vi "Experiment01.vi"() -> ()   [LabVIEW 2009]
uses:
  <vilib>/imath/engines/lvmath2/RunTimeEngine/ErrorHandling/NIMS_Finalize Error.vi
  <vilib>/imath/engines/lvmath2/RunTimeEngine/Parser/MC_Version.vi
  <vilib>/imath/engines/lvmath2/RunTimeEngine/NodeEndStatement/NIMS_NodeEndStatement_Output.vi
  <instcachedir>/0/NIMS_NodeEndStatement_Output_B70DDD75627E4997AAE11E9955EDAA25.lvgen/NIMS_NodeEndStatement_Output_B70DDD75627E4997AAE11E9955EDAA25_002.vi
  <instcachedir>/0/NIMS_NodeEndStatement_Output_B70DDD75627E4997AAE11E9955EDAA25.lvgen/NIMS_NodeEndStatement_Output_B70DDD75627E4997AAE11E9955EDAA25_003.vi
  <vilib>/imath/engines/lvmath/Functions/Error Handling/MergeErrorsWrapper.vi
  <instcachedir>/0/NIMS_NodeEndStatement_Output_B70DDD75627E4997AAE11E9955EDAA25.lvgen/NIMS_NodeEndStatement_Output_B70DDD75627E4997AAE11E9955EDAA25_001.vi
  <vilib>/imath/engines/lvmath2/RunTimeEngine/Managers/WorkSpace/UID Generator.vi
  <vilib>/imath/engines/lvmath/Functions/Error Handling/error.ctl
  <instcachedir>/0/NIMS_NodeEndStatement_Output_B70DDD75627E4997AAE11E9955EDAA25.lvgen/NIMS_NodeEndStatement_Output_B70DDD75627E4997AAE11E9955EDAA25_000.vi
  <vilib>/imath/engines/lvmath2/RunTimeEngine/Managers/SymbolTable/Clear UID.vi
  <vilib>/imath/engines/lvmath2/RunTimeEngine/VariableToken/NIMS_VariableToken_CondDefined.vi
  <instcachedir>/0/NIMS_VariableToken_CondDefined_5641E79000FB4D628475532441475385.lvgen/NIMS_VariableToken_CondDefined_5641E79000FB4D628475532441475385_001.vi
  <vilib>/imath/engines/lvmath/Functions/Error Handling/MC_Mask_Errors.vi
  <vilib>/imath/engines/lvmath2/RunTimeEngine/BuiltInFunctions/rem/NIMS_rem_no checks.vi
  <instcachedir>/0/NIMS_rem_no checks_4CC9B305AB7E42EF90AFC4973FB32F8D.lvgen/NIMS_rem_no checks_4CC9B305AB7E42EF90AFC4973FB32F8D_000.vi
  <vilib>/imath/engines/lvmath2/RunTimeEngine/BuiltInFunctions/uint32/NIMS_uint32(real).vi
  <instcachedir>/0/NIMS_uint32(real)_FDC83D68D45943DDB8F3F934FF8A712F.lvgen/NIMS_uint32(real)_FDC83D68D45943DDB8F3F934FF8A712F_000.vi
  <vilib>/imath/engines/lvmath2/RunTimeEngine/BuiltInFunctions/double/NIMS_double.vi
  <instcachedir>/0/NIMS_double_2CE444F3CE4146B199A482FE12545E45.lvgen/NIMS_double_2CE444F3CE4146B199A482FE12545E45_000.vi
  <vilib>/imath/engines/lvmath2/RunTimeEngine/RangeToken/NIMS_Range.vi
  <instcachedir>/0/NIMS_Range_6D647EC16A744C98B5DE1D649A2D648D.lvgen/NIMS_Range_6D647EC16A744C98B5DE1D649A2D648D_001.vi
  <vilib>/imath/engines/lvmath2/RunTimeEngine/BuiltInFunctions/length/NIMS_length(GV).vi
  <instcachedir>/0/NIMS_length(GV)_7D6E94E728E145E68721C53861296D96.lvgen/NIMS_length(GV)_7D6E94E728E145E68721C53861296D96_000.vi
  <instcachedir>/0/NIMS_Range_6D647EC16A744C98B5DE1D649A2D648D.lvgen/NIMS_Range_6D647EC16A744C98B5DE1D649A2D648D_000.vi
  <vilib>/imathl/engines/lvmath/Functions/Error Handling/Create Error.vi
  <vilib>/imath/engines/lvmath2/RunTimeEngine/ReplaceToken/NIMS_Replace - V(S)=S.vi
  <instcachedir>/0/NIMS_Replace - V(S)=S_670A9E0533664C1D848C8E58B3321B6A.lvgen/NIMS_Replace - V(S)=S_670A9E0533664C1D848C8E58B3321B6A_002.vi
  <vilib>/imath/engines/lvmath2/RunTimeEngine/ReplaceToken/NIMS_Replace - Size Check _(_)=S.vi
  <instcachedir>/0/NIMS_Replace - Size Check _(_)=S_8596181D73404097BAB9CBB006194BB0.lvgen/NIMS_Replace - Size Check _(_)=S_8596181D73404097BAB9CBB006194BB0_002.vi
  <vilib>/imath/engines/lvmath2/RunTimeEngine/ReplaceToken/NIMS_Replace - Check Linear.vi
  <instcachedir>/0/NIMS_Replace - Check Linear_9243CBB174894FF6977027453DA6955E.lvgen/NIMS_Replace - Check Linear_9243CBB174894FF6977027453DA6955E_002.vi
  <vilib>/imath/engines/lvmath2/RunTimeEngine/VariableToken/NIMS_VariableToken_CondDefinedDefinedByReplace.vi
  <instcachedir>/0/NIMS_VariableToken_CondDefinedDefinedByReplace_D162CFFC24174562A9FEA619A91E1A56.lvgen/NIMS_VariableToken_CondDefinedDefinedByReplace_D162CFFC24174562A9FEA619A91E1A56_002.vi
  <vilib>/imath/engines/lvmath2/RunTimeEngine/CommandStatement/MC_CommandStatement_break.vi
  <vilib>/imath/engines/lvmath2/RunTimeEngine/LocalVariableDefStatement/MC_LocalVariableDefStatement_Display.vi
  <vilib>/imath/engines/lvmath2/RunTimeEngine/RunTimeType/NIMS_RunTimeType_From StrictType (excl LVString).vi
  <vilib>/imath/engines/lvmath2/RunTimeEngine/ArithmeticOperatorToken/NIMS_ArithmeticOperator_times.vi
  <instcachedir>/0/NIMS_ArithmeticOperator_times_3987BC660D7947CD8628C10658A43225.lvgen/NIMS_ArithmeticOperator_times_3987BC660D7947CD8628C10658A43225_001.vi
  <instcachedir>/0/NIMS_ArithmeticOperator_times_3987BC660D7947CD8628C10658A43225.lvgen/NIMS_ArithmeticOperator_times_3987BC660D7947CD8628C10658A43225_000.vi
  <vilib>/imath/engines/lvmath2/RunTimeEngine/VariableToken/Read/NIMS_Get Elements - RV(_) - Check.vi
  <instcachedir>/0/NIMS_Get Elements - RV(_) - Check_60F12861D0564803969A5D0D0D1716CD.lvgen/NIMS_Get Elements - RV(_) - Check_60F12861D0564803969A5D0D0D1716CD_000.vi
  <instcachedir>/0/NIMS_VariableToken_CondDefined_5641E79000FB4D628475532441475385.lvgen/NIMS_VariableToken_CondDefined_5641E79000FB4D628475532441475385_000.vi
  <instcachedir>/0/NIMS_VariableToken_CondDefined_5641E79000FB4D628475532441475385.lvgen/NIMS_VariableToken_CondDefined_5641E79000FB4D628475532441475385_003.vi
  <vilib>/imath/engines/lvmath2/RunTimeEngine/BuiltInFunctions/abs/NIMS_abs(signed).vi
  <instcachedir>/0/NIMS_abs(signed)_C4FCB8E6058B49B797C7C8D53CA5F6EC.lvgen/NIMS_abs(signed)_C4FCB8E6058B49B797C7C8D53CA5F6EC_000.vi
  <instcachedir>/0/NIMS_Replace - V(S)=S_670A9E0533664C1D848C8E58B3321B6A.lvgen/NIMS_Replace - V(S)=S_670A9E0533664C1D848C8E58B3321B6A_001.vi
  <instcachedir>/0/NIMS_Replace - Size Check _(_)=S_8596181D73404097BAB9CBB006194BB0.lvgen/NIMS_Replace - Size Check _(_)=S_8596181D73404097BAB9CBB006194BB0_001.vi
  <instcachedir>/0/NIMS_Replace - Check Linear_9243CBB174894FF6977027453DA6955E.lvgen/NIMS_Replace - Check Linear_9243CBB174894FF6977027453DA6955E_001.vi
  <instcachedir>/0/NIMS_VariableToken_CondDefinedDefinedByReplace_D162CFFC24174562A9FEA619A91E1A56.lvgen/NIMS_VariableToken_CondDefinedDefinedByReplace_D162CFFC24174562A9FEA619A91E1A56_001.vi
  <instcachedir>/0/NIMS_Replace - V(S)=S_670A9E0533664C1D848C8E58B3321B6A.lvgen/NIMS_Replace - V(S)=S_670A9E0533664C1D848C8E58B3321B6A_000.vi
  <instcachedir>/0/NIMS_Replace - Size Check _(_)=S_8596181D73404097BAB9CBB006194BB0.lvgen/NIMS_Replace - Size Check _(_)=S_8596181D73404097BAB9CBB006194BB0_000.vi
  <instcachedir>/0/NIMS_Replace - Check Linear_9243CBB174894FF6977027453DA6955E.lvgen/NIMS_Replace - Check Linear_9243CBB174894FF6977027453DA6955E_000.vi
  <instcachedir>/0/NIMS_VariableToken_CondDefinedDefinedByReplace_D162CFFC24174562A9FEA619A91E1A56.lvgen/NIMS_VariableToken_CondDefinedDefinedByReplace_D162CFFC24174562A9FEA619A91E1A56_000.vi
  <vilib>/imath/engines/lvmath2/RunTimeEngine/Managers/SymbolTable/NIMS_WorkSpace.lvlib
panel:
  out "Current VI path 11":string
  out "New Path for Picture 11":string
  out "Part Stripped 11":string
  out "Stripped Path 11":string
  out "Current VI path 10":string
  out "New Path for Picture 10":string
  out "Part Stripped 10":string
  out "Stripped Path 10":string
  out "Current VI path 9":string
  out "New Path for Picture 9":string
  out "Part Stripped 9":string
  out "Stripped Path 9":string
  out "Current VI path 8":string
  out "New Path for Picture 8":string
  out "Part Stripped 8":string
  out "Stripped Path 8":string
  out "Current VI path 7":string
  out "New Path for Picture 7":string
  out "Part Stripped 7":string
  out "Stripped Path 7":string
  out "Current VI path 6":string
  out "New Path for Picture 6":string
  out "Part Stripped 6":string
  out "Stripped Path 6":string
  out "Current VI path 5":string
  out "New Path for Picture 5":string
  out "Part Stripped 5":string
  out "Stripped Path 5":string
  out "Current VI path 4":string
  out "New Path for Picture 4":string
  out "Part Stripped 4":string
  out "Stripped Path 4":string
  out "Current VI path 3":string
  out "New Path for Picture 3":string
  out "Part Stripped 3":string
  out "Stripped Path 3":string
  out "Current VI path 2":string
  out "New Path for Picture 2":string
  out "Part Stripped 2":string
  out "Stripped Path 2":string
  out "Current VI path":string
  out "New Path for Picture":string
  out "Part Stripped":string
  out "Stripped Path":string
  out "error out":errorcluster
  in  "2.TECNIQUE USED TO CALCULATE VSWR":bool
  out "error out":errorcluster
  in  "1.TECNIQUE USED TO CALCULATE VSWR":bool
  out "?":errorcluster
  out "?":errorcluster
  in  "?":T1(tab)
  out "?":dbl[](graph)
  out "Characteristic Impedance":dbl
  out "Voltage 2":dbl
  out "Distance(Meter)":dbl
  in  "Slide":dbl(slide) scale=0.0..0.3
  out "?":errorcluster
  in  "HELP FOR SLOTTED LINE":bool
  out "error out":errorcluster
  out "?":dbl[](graph)
  out "VSWR Meter":dbl(knob) caption="Meter" scale=500.0..1.0 scale format="%#_10g"
  out "Ideal VSWR":dbl
  in  "?":enum32{"LOADS"}(tab)
  in  "Type of Loads":T2(radio)
  out "Resistance":dbl
  out "Reactance":dbl
  in  "Resistance":dbl(slide) scale=0.0..1000.0
  in  "Reactance":dbl(slide) scale=0.0..1000.0
  out "?":errorcluster
  in  "HELP FOR LOADS":bool
  out "error out":errorcluster
  in  "?":enum32{"ATTENUATOR"}(tab)
  out "?":dbl[](graph)
  in  "Set the value of attenuation in dB":dbl(slide) scale=0.0..100.0
  out "?":errorcluster
  in  "HELP FOR ATTENUATOR":bool
  out "error out":errorcluster
  in  "?":enum32{"ISOLATOR"}(tab)
  out "?":dbl[](graph)
  in  "?":bool
  out "?":errorcluster
  in  "HELP FOR ISOLATOR":bool
  out "error out":errorcluster
  in  "?":enum32{"MODULATOR"}(tab)
  in  "Modulating Frequency(KHz)":dbl(slide) scale=0.5..1.5
  out "?":errorcluster
  out "?":dbl[](graph)
  in  "HELP FOR MODULATOR":bool
  out "error out":errorcluster
  in  "?":enum32{"SOURCE"}(tab)
  out "?":dbl[](graph)
  in  "Frequency of carrier wave(GHz)":dbl(slide) scale=8.0..15.0
  in  "Voltage":dbl(knob) scale=0.0..20.0 scale format="%#_10g"
  out "?":errorcluster
  in  "HELP FOR SOURCE":bool
  out "error out":errorcluster
  # "Backward Direction"
  # "Forward direction"
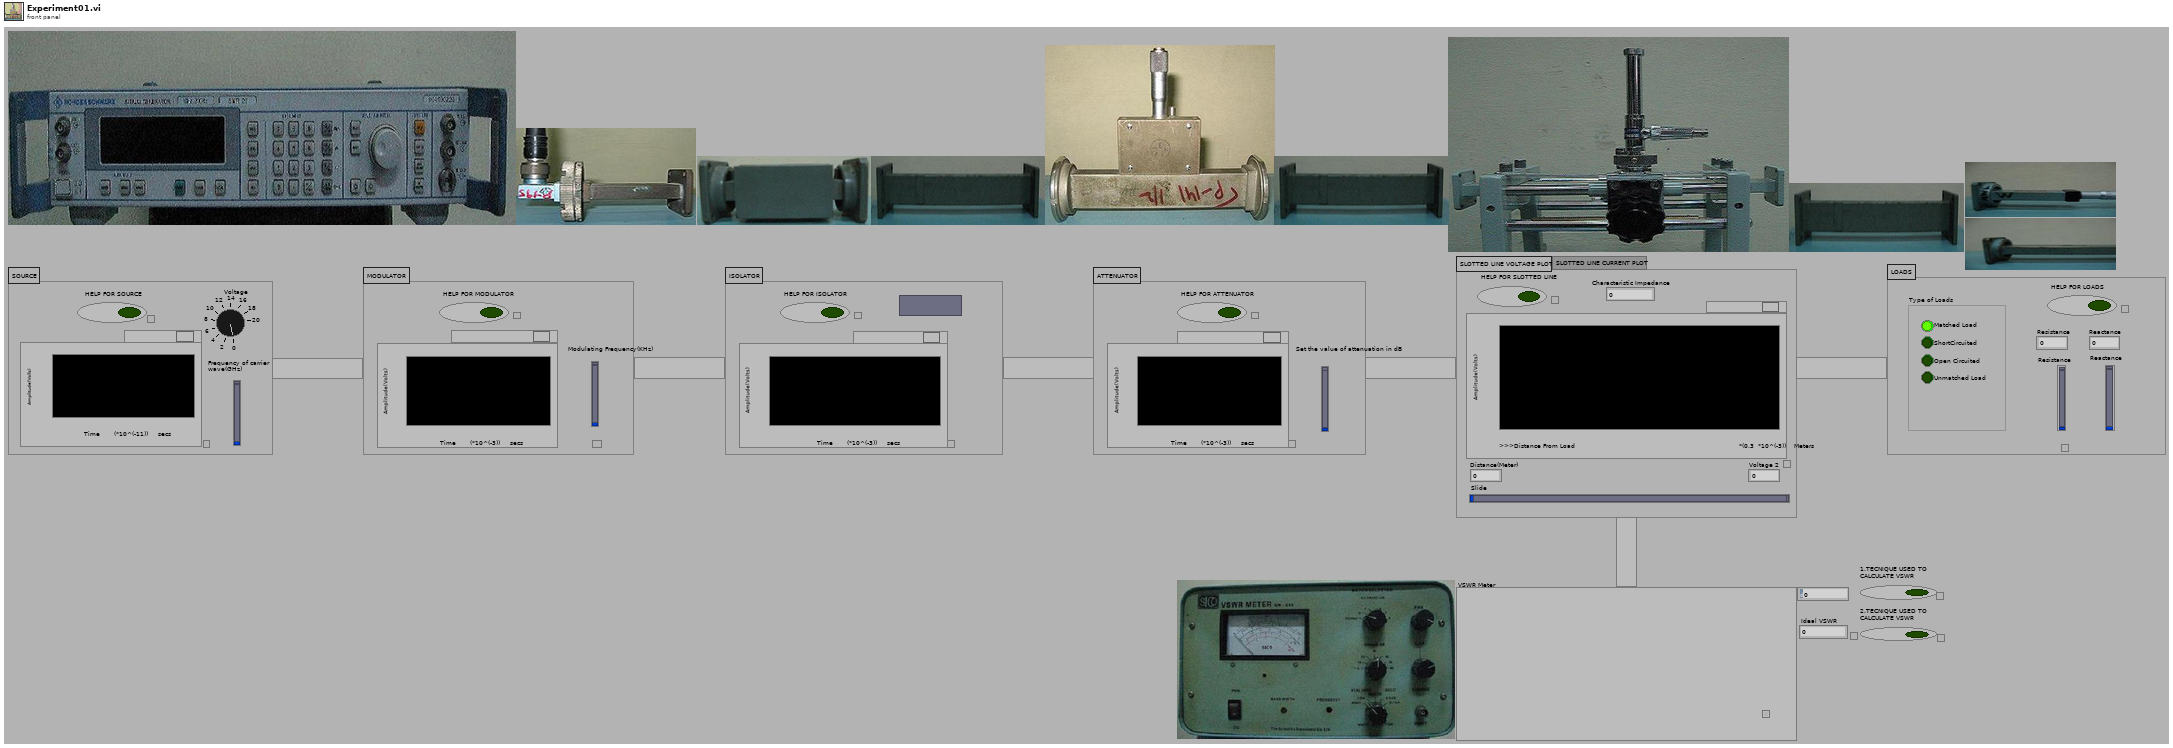
[diagram p1: front panel]
types:
  T1 = enum32{"SLOTTED LINE VOLTAGE PLOT", "SLOTTED LINE CURRENT PLOT"}
  T2 = enum32{"Matched Load", "ShortCircuited", "Open Circuited", "Unmatched Load"}
  T3 = typedef "imagedata.ctl" = cluster{"image type":i32, "image depth":i32, "image":u8[], "mask":u8[], "colors":u32[], "Rectangle":cluster{"left":i16, "top":i16, "right":i16, "bottom":i16}}
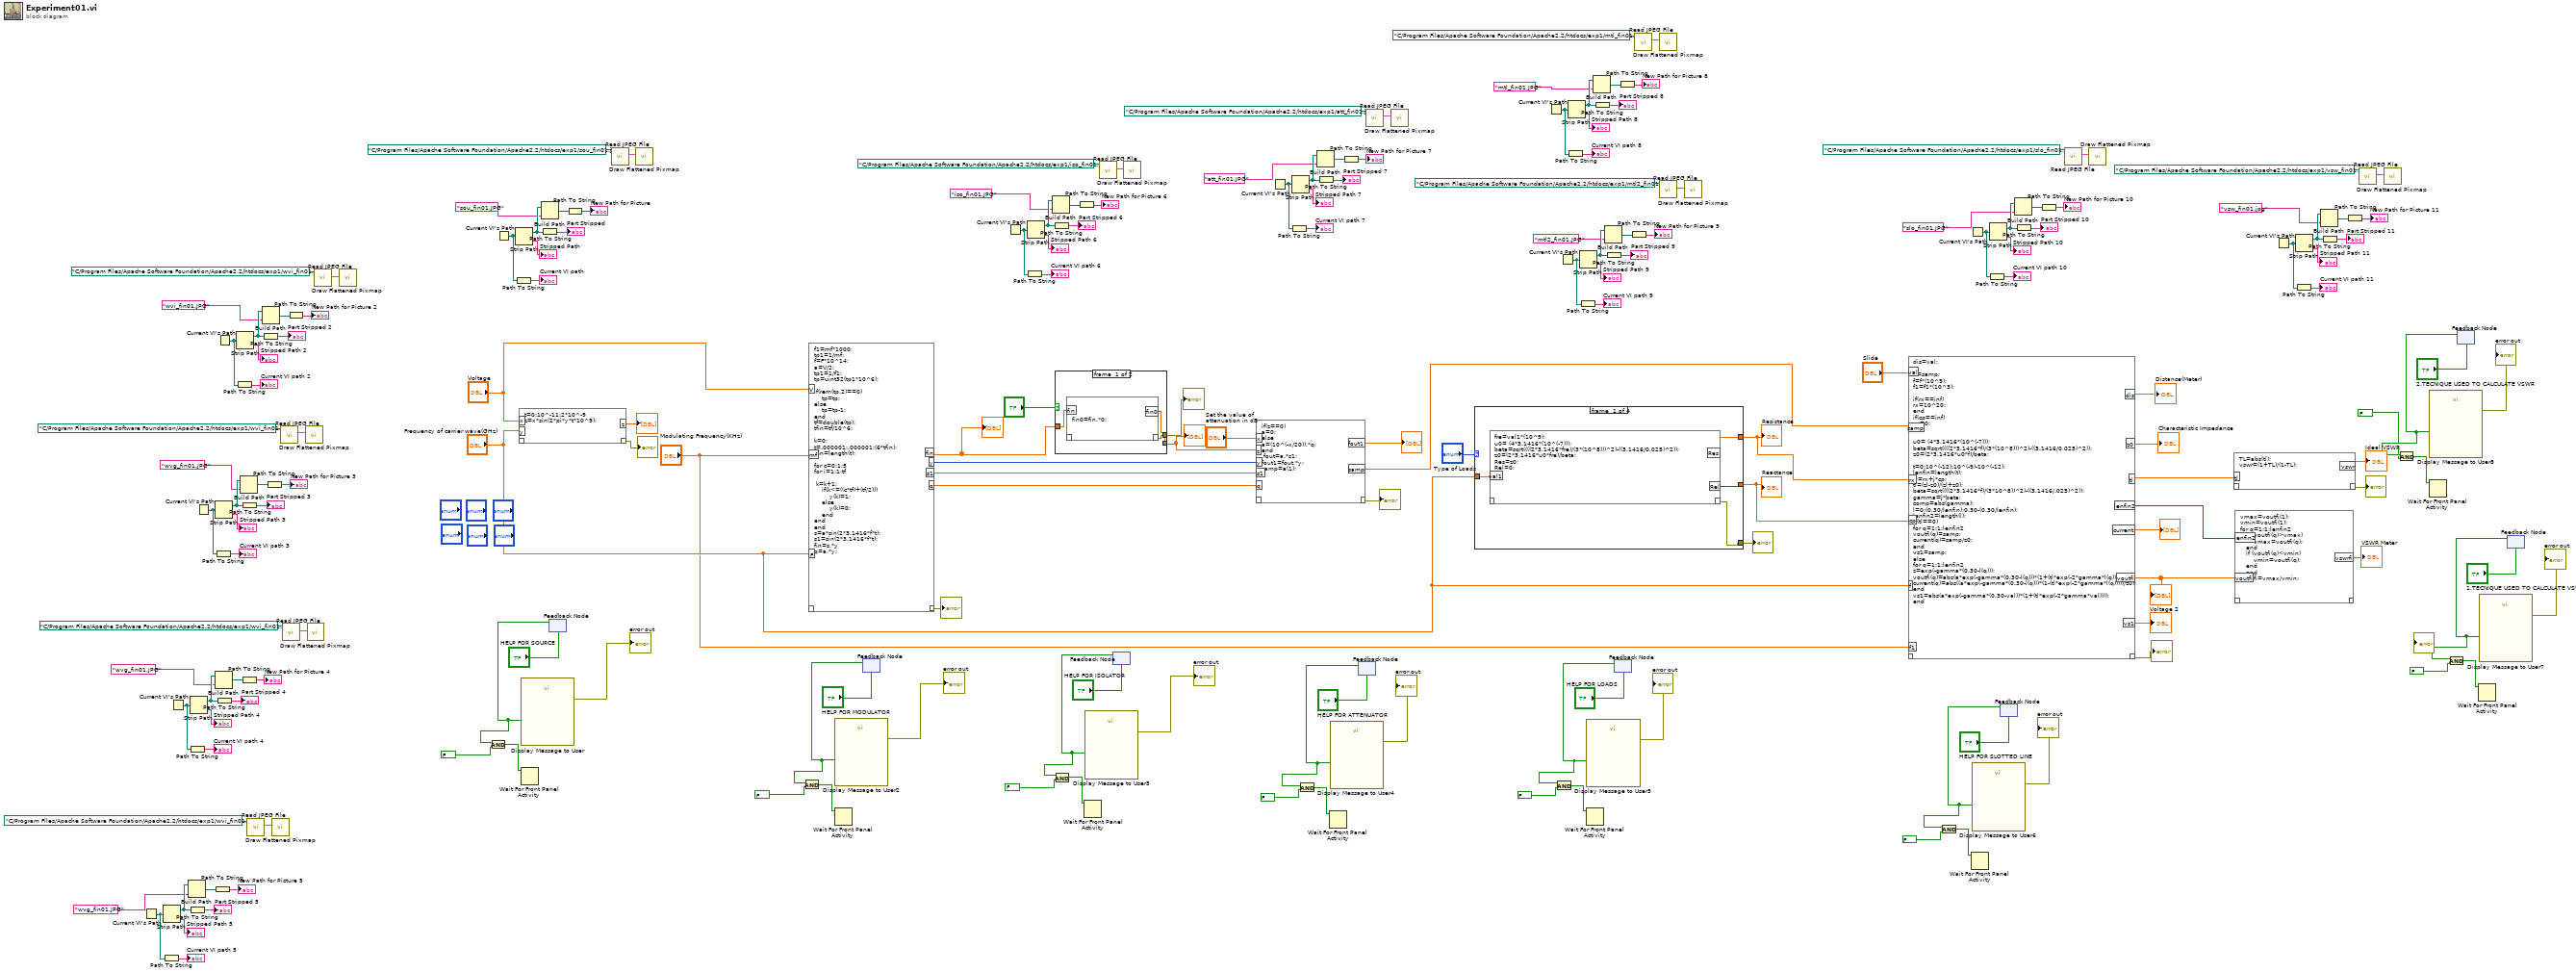
[diagram p0: block diagram]
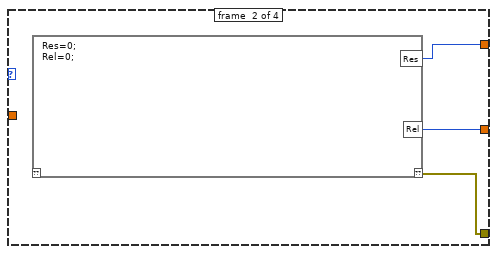
[diagram p2: hidden frame]
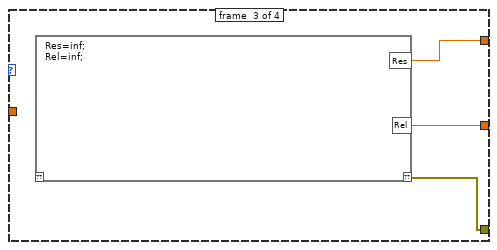
[diagram p3: hidden frame]
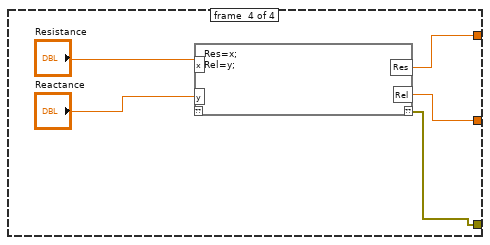
[diagram p4: hidden frame]
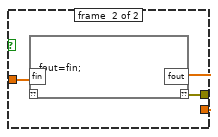
[diagram p5: hidden frame]
diagram:
  n1 = Current VI's Path() -> (path=w78:path)
  n2 = Path To String(path=w78) -> (string=→"Current VI path 5":string)
  n3 = Strip Path(path=w78) -> (stripped path=w82:path, name=→"Stripped Path 5":string)
  n4 = Current VI's Path() -> (path=w86:path)
  n5 = Build Path(base path=w82, name or relative path="wvg_fin01.JPG") -> (appended path=w75:path)
  n6 = Path To String(path=w82) -> (string=→"Part Stripped 5":string)
  n7 = Path To String(path=w86) -> (string=→"Current VI path 4":string)
  n8 = Strip Path(path=w86) -> (stripped path=w90:path, name=→"Stripped Path 4":string)
  n9 = Current VI's Path() -> (path=w94:path)
  n10 = Path To String(path=w75) -> (string=→"New Path for Picture 5":string)
  n11 = Path To String(path=w94) -> (string=→"Current VI path 3":string)
  n12 = Build Path(base path=w90, name or relative path="wvg_fin01.JPG") -> (appended path=w83:path)
  n13 = Strip Path(path=w94) -> (stripped path=w98:path, name=→"Stripped Path 3":string)
  n14 = Path To String(path=w90) -> (string=→"Part Stripped 4":string)
  n15 = Current VI's Path() -> (path=w102:path)
  n16 = Path To String(path=w102) -> (string=→"Current VI path 2":string)
  n17 = Strip Path(path=w102) -> (stripped path=w106:path, name=→"Stripped Path 2":string)
  n18 = Build Path(base path=w98, name or relative path="wvg_fin01.JPG") -> (appended path=w91:path)
  n19 = Path To String(path=w83) -> (string=→"New Path for Picture 4":string)
  n20 = Path To String(path=w98) -> (string=→"Part Stripped 3":string)
  n21 = call <vilib>:"Read JPEG File.vi"("path to JPEG file"=path "C:/Program Files/Apache Software Foundation/Apache2.2/htdocs/exp1/wvi_fin01.jpg") -> ("image data"=w107:T3)  [unwired: 1 in, 9 out]
  n22 = Build Path(base path=w106, name or relative path="wvi_fin01.JPG") -> (appended path=w99:path)
  n23 = Path To String(path=w106) -> (string=→"Part Stripped 2":string)
  n24 = Path To String(path=w91) -> (string=→"New Path for Picture 3":string)
  n25 = call <vilib>:"Draw Flattened Pixmap.vi"("image data"=w107) -> ()  [unwired: 1 in, 8 out]
  n26 = call <vilib>:"Read JPEG File.vi"("path to JPEG file"=path "C:/Program Files/Apache Software Foundation/Apache2.2/htdocs/exp1/wvi_fin01.jpg") -> ("image data"=w109:T3)  [unwired: 1 in, 9 out]
  n27 = call <vilib>:"Read JPEG File.vi"("path to JPEG file"=path "C:/Program Files/Apache Software Foundation/Apache2.2/htdocs/exp1/wvi_fin01.jpg") -> ("image data"=w108:T3)  [unwired: 1 in, 9 out]
  n28 = Path To String(path=w99) -> (string=→"New Path for Picture 2":string)
  n29 = call <vilib>:"Draw Flattened Pixmap.vi"("image data"=w109) -> ()  [unwired: 1 in, 8 out]
  n30 = call <vilib>:"Draw Flattened Pixmap.vi"("image data"=w108) -> ()  [unwired: 1 in, 8 out]
  n31 = call <vilib>:"Read JPEG File.vi"("path to JPEG file"=path "C:/Program Files/Apache Software Foundation/Apache2.2/htdocs/exp1/wvi_fin01.jpg") -> ("image data"=w110:T3)  [unwired: 1 in, 9 out]
  n32 = call <vilib>:"Draw Flattened Pixmap.vi"("image data"=w110) -> ()  [unwired: 1 in, 8 out]
  n33 = Current VI's Path() -> (path=w64:path)
  n34 = Path To String(path=w64) -> (string=→"Current VI path":string)
  n35 = Strip Path(path=w64) -> (stripped path=w68:path, name=→"Stripped Path":string)
  n36 = mathscript code="t=0:10^-11:2*10^-9\nz=x*sin(2*pi*y*t*10^9);"("x"="Voltage", "y"="Frequency of carrier wave(GHz)") -> ("??"=→"?":errorcluster, "z"=→"?":dbl[])  [unwired: 1 in]
  n37 = Build Path(base path=w68, name or relative path="sou_fin01.JPG" ("name or relative path 2")) -> (appended path=w61:path)
  n38 = Path To String(path=w68) -> (string=→"Part Stripped":string)
  n39 = feedback #1("HELP FOR SOURCE") -> (w186:bool)
  n40 = And(x=w186, y=FALSE) -> (x .and. y?=w184:bool)
  n41 = Wait For Front Panel Activity(3:w184) -> ()  [unwired: 3 out]
  n42 = call "Display Message to User"("Enable"=w186) -> ("error out"=→"error out":errorcluster, "CLOSE"=w188:bool)  [unwired: 2 in, 7 out]
  n43 = Path To String(path=w61) -> (string=→"New Path for Picture":string)
  n44 = call <vilib>:"Read JPEG File.vi"("path to JPEG file"=path "C:/Program Files/Apache Software Foundation/Apache2.2/htdocs/exp1/sou_fin01.jpg") -> ("image data"=w70:T3)  [unwired: 1 in, 9 out]
  n45 = call <vilib>:"Draw Flattened Pixmap.vi"("image data"=w70) -> ()  [unwired: 1 in, 8 out]
  n46 = mathscript code="f1=mf*1000;\ntp1=1/mf;\nf=F*10^14;\na=V/2;\ntp1=1/f1;\ntp=uint32(tp1*10^6);\n\nif(rem(tp,2)==0)\n    tp=tp;\nelse\n    tp=tp-1;\nend\ntf=double(tp);\ntfin=tf/10^6;\n\nk=0;\nt=.000001:.000001:(6*tfin);\nlen=length(t);\n\nfor c=0:1:5\nfor i=1:1:tf\n  \n k=k+1;\n    if(k<=((c*tf)+(tf/2)))\n        y(k)=1;\n    else\n        y(k)=0;\n    end\nend\nend\ns=a*sin(2*3.1416*f*t);\ns1=sin(2*3.1416*f*t);\nfin=s.*y\nq=a.*y;"("V"="Voltage", "mf"="Modulating Frequency(KHz)", "F"="Frequency of carrier wave(GHz)") -> ("??"=→"?":errorcluster, "fin"=w138:dbl[], "s1"=w133:dbl[], "q"=w132:dbl[], "y"=w134:i32[])  [unwired: 1 in]
  "?" <- w138
  n47 = feedback #2("HELP FOR MODULATOR") -> (w180:bool)
  n48 = And(x=w180, y=FALSE) -> (x .and. y?=w178:bool)
  n49 = Wait For Front Panel Activity(3:w178) -> ()  [unwired: 3 out]
  n50 = call "Display Message to User2"("Enable"=w180) -> ("error out"=→"error out":errorcluster, "CLOSE"=w182:bool)  [unwired: 2 in, 7 out]
  n51 = Current VI's Path() -> (path=w51:path)
  n52 = Path To String(path=w51) -> (string=→"Current VI path 6":string)
  n53 = Strip Path(path=w51) -> (stripped path=w55:path, name=→"Stripped Path 6":string)
  n54 = Build Path(base path=w55, name or relative path="iso_fin01.JPG") -> (appended path=w48:path)
  n55 = Path To String(path=w55) -> (string=→"Part Stripped 6":string)
  n56 = case shown="False" "?" {
    tunnel: [w193 w214] -> w135
    tunnel: w138 -> [w194 w215]
    tunnel: [w192 w213] -> w112
    frame #0 {
      n57 = mathscript code="fin0=fin.*0;"("fin"=w194) -> ("??"=w192:errorcluster, "fin0"=w193:dbl[])  [unwired: 1 in]
    }
    frame #1 {
      n58 = mathscript code="fout=fin;"("fin"=w215) -> ("??"=w213:errorcluster, "fout"=w214:dbl[])  [unwired: 1 in]
    }
  }
  "?" <- w135
  "?" <- w112
  n59 = Path To String(path=w48) -> (string=→"New Path for Picture 6":string)
  n60 = call <vilib>:"Read JPEG File.vi"("path to JPEG file"=path "C:/Program Files/Apache Software Foundation/Apache2.2/htdocs/exp1/iso_fin01.jpg") -> ("image data"=w59:T3)  [unwired: 1 in, 9 out]
  n61 = feedback #3("HELP FOR ISOLATOR") -> (w174:bool)
  n62 = And(x=w174, y=FALSE) -> (x .and. y?=w172:bool)
  n63 = Wait For Front Panel Activity(3:w172) -> ()  [unwired: 3 out]
  n64 = call "Display Message to User3"("Enable"=w174) -> ("error out"=→"error out":errorcluster, "CLOSE"=w176:bool)  [unwired: 2 in, 7 out]
  n65 = call <vilib>:"Draw Flattened Pixmap.vi"("image data"=w59) -> ()  [unwired: 1 in, 8 out]
  n66 = mathscript code="if(z==0)\na=0; \nelse\na=(10^(-x/20)).*q;\nend\n fout=a.*s1;\nfout1=fout.*y;\nsamp=a(1);"("x"="Set the value of attenuation in dB", "z"=w135, "y"=w134, "s1"=w133, "q"=w132) -> ("??"=→"?":errorcluster, "fout1"=→"?":dbl[], "samp"=w127:dbl)  [unwired: 1 in]
  n67 = Current VI's Path() -> (path=w43:path)
  n68 = Path To String(path=w43) -> (string=→"Current VI path 7":string)
  n69 = Strip Path(path=w43) -> (stripped path=w47:path, name=→"Stripped Path 7":string)
  n70 = Build Path(base path=w47, name or relative path="att_fin01.JPG") -> (appended path=w40:path)
  n71 = Path To String(path=w47) -> (string=→"Part Stripped 7":string)
  n72 = Path To String(path=w40) -> (string=→"New Path for Picture 7":string)
  n73 = feedback #4("HELP FOR ATTENUATOR") -> (w168:bool)
  n74 = And(x=w168, y=FALSE) -> (x .and. y?=w166:bool)
  n75 = Wait For Front Panel Activity(3:w166) -> ()  [unwired: 3 out]
  n76 = call "Display Message to User4"("Enable"=w168) -> ("error out"=→"error out":errorcluster, "CLOSE"=w170:bool)  [unwired: 2 in, 7 out]
  n77 = call <vilib>:"Read JPEG File.vi"("path to JPEG file"=path "C:/Program Files/Apache Software Foundation/Apache2.2/htdocs/exp1/att_fin01.jpg") -> ("image data"=w60:T3)  [unwired: 1 in, 9 out]
  n78 = call <vilib>:"Draw Flattened Pixmap.vi"("image data"=w60) -> ()  [unwired: 1 in, 8 out]
  n79 = case shown="\"Unmatched Load\"" "Type of Loads" {
    tunnel: "Frequency of carrier wave(GHz)" -> [w235 _ _ _]
    tunnel: [w233 w321 w347 w374] -> w126
    tunnel: [w234 w322 w348 w373] -> w125
    tunnel: [w232 w320 w346 w372] -> w111
    frame #0 {
      n80 = mathscript code="fre=val1*(10^9);\nu0= (4*3.1416*(10^(-7)));\nbeta=sqrt((((2*3.1416*fre)/(3*(10^8)))^2)-((3.1416/0.025)^2));\nz0=(2*3.1416*u0*fre)/beta;\nRes=z0;\nRel=0;"("val1"=w235) -> ("??"=w232:errorcluster, "Rel"=w234:i32, "Res"=w233:cdb)  [unwired: 1 in]
    }
    frame #1 {
      n81 = mathscript code="Res=0;\nRel=0;"() -> ("??"=w320:errorcluster, "Res"=w321:i32, "Rel"=w322:i32)  [unwired: 1 in]
    }
    frame #2 {
      n82 = mathscript code="Res=inf;\nRel=inf;"() -> ("??"=w346:errorcluster, "Res"=w347:dbl, "Rel"=w348:dbl)  [unwired: 1 in]
    }
    frame #3 {
      n83 = mathscript code="Res=x;\nRel=y;"("x"="Resistance", "y"="Reactance") -> ("??"=w372:errorcluster, "Res"=w374:dbl, "Rel"=w373:dbl)  [unwired: 1 in]
    }
  }
  "Resistance" <- w126
  "Reactance" <- w125
  "?" <- w111
  n84 = Current VI's Path() -> (path=w34:path)
  n85 = Current VI's Path() -> (path=w26:path)
  n86 = Path To String(path=w34) -> (string=→"Current VI path 8":string)
  n87 = Strip Path(path=w34) -> (stripped path=w39:path, name=→"Stripped Path 8":string)
  n88 = Path To String(path=w26) -> (string=→"Current VI path 9":string)
  n89 = Strip Path(path=w26) -> (stripped path=w31:path, name=→"Stripped Path 9":string)
  n90 = Build Path(base path=w39, name or relative path="mtl_fin01.JPG") -> (appended path=w32:path)
  n91 = Path To String(path=w39) -> (string=→"Part Stripped 8":string)
  n92 = Build Path(base path=w31, name or relative path="mtl2_fin01.JPG") -> (appended path=w24:path)
  n93 = Path To String(path=w31) -> (string=→"Part Stripped 9":string)
  n94 = feedback #5("HELP FOR LOADS") -> (w162:bool)
  n95 = And(x=w162, y=FALSE) -> (x .and. y?=w160:bool)
  n96 = Wait For Front Panel Activity(3:w160) -> ()  [unwired: 3 out]
  n97 = call "Display Message to User5"("Enable"=w162) -> ("error out"=→"error out":errorcluster, "CLOSE"=w164:bool)  [unwired: 2 in, 7 out]
  n98 = Path To String(path=w32) -> (string=→"New Path for Picture 8":string)
  n99 = Path To String(path=w24) -> (string=→"New Path for Picture 9":string)
  n100 = call <vilib>:"Read JPEG File.vi"("path to JPEG file"=path "C:/Program Files/Apache Software Foundation/Apache2.2/htdocs/exp1/mtl_fin01.jpg") -> ("image data"=w2:T3)  [unwired: 1 in, 9 out]
  n101 = call <vilib>:"Draw Flattened Pixmap.vi"("image data"=w2) -> ()  [unwired: 1 in, 8 out]
  n102 = call <vilib>:"Read JPEG File.vi"("path to JPEG file"=path "C:/Program Files/Apache Software Foundation/Apache2.2/htdocs/exp1/mtl2_fin01.jpg") -> ("image data"=w57:T3)  [unwired: 1 in, 9 out]
  n103 = call <vilib>:"Draw Flattened Pixmap.vi"("image data"=w57) -> ()  [unwired: 1 in, 8 out]
  n104 = mathscript code="dis=val;\n\na=samp;\nf=f*(10^9);\nf1=f1*(10^3);\n\nif(rx==inf)\nrx=10^20;\nend\nif(cp==inf)\ncp=0;\nend\n\nu0= (4*3.1416*(10^(-7)));\nbeta=sqrt((((2*3.1416*f)/(3*(10^8)))^2)-((3.1416/0.025)^2));\nz0=(2*3.1416*u0*f)/beta;\n\nt=0:10^(-12):10^(-9)-10^(-12);\nlenfin=length(t);\nzl=rx+j*cp;\ntl=(zl-z0)/(zl+z0);\nbeta=sqrt((((2*3.1416*f)/(3*10^8))^2)-((3.1416/.025)^2));\ngamma=j*beta;\ncomp=abs(gamma);\nl=0:(0.30/lenfin):0.30-(0.30/lenfin);\nlenfin2=length(l);\nif(tl==0)\nfor q=1:1:lenfin2\nvoutfi(q)=samp;\ncurrent(q)=samp/z0;\nend\nvs1=samp;\nelse\nfor q=1:1:lenfin2\nz=exp(-gamma*(0.30-l(q)));\nvoutfi(q)=abs(a*exp(-gamma*(0.30-l(q)))*(1+(tl*exp(-2*gamma*l(q)))));\ncurrent(q)=abs((a*exp(-gamma*(0.30-l(q)))*(1-(tl*exp(-2*gamma*l(q)))))/z0);\nend\nvs1=abs(a*exp(-gamma*(0.30-val))*(1+(tl*exp(-2*gamma*val))));\nend"("val"="Slide", "samp"=w127, "rx"=w126, "cp"=w125, "f"="Frequency of carrier wave(GHz)", "f1"="Modulating Frequency(KHz)") -> ("??"=→"?":errorcluster, "dis"=→"Distance(Meter)":dbl, "z0"=→"Characteristic Impedance":cdb, "tl"=w115:cdb, "lenfin2"=w120:i32, "current"=→"?":cdb[], "voutfi"=w118:dbl[], "vs1"=→"Voltage 2":dbl)  [unwired: 1 in]
  "?" <- w118
  n105 = Current VI's Path() -> (path=w18:path)
  n106 = Path To String(path=w18) -> (string=→"Current VI path 10":string)
  n107 = Strip Path(path=w18) -> (stripped path=w23:path, name=→"Stripped Path 10":string)
  n108 = feedback #6("HELP FOR SLOTTED LINE") -> (w156:bool)
  n109 = And(x=w156, y=FALSE) -> (x .and. y?=w154:bool)
  n110 = Wait For Front Panel Activity(3:w154) -> ()  [unwired: 3 out]
  n111 = call "Display Message to User6"("Enable"=w156) -> ("error out"=→"error out":errorcluster, "CLOSE"=w158:bool)  [unwired: 2 in, 7 out]
  n112 = Build Path(base path=w23, name or relative path="slo_fin01.JPG") -> (appended path=w16:path)
  n113 = Path To String(path=w23) -> (string=→"Part Stripped 10":string)
  n114 = Path To String(path=w16) -> (string=→"New Path for Picture 10":string)
  n115 = call <vilib>:"Read JPEG File.vi"("path to JPEG file"=path "C:/Program Files/Apache Software Foundation/Apache2.2/htdocs/exp1/slo_fin01.jpg") -> ("image data"=w58:T3)  [unwired: 1 in, 9 out]
  n116 = call <vilib>:"Draw Flattened Pixmap.vi"("image data"=w58) -> ()  [unwired: 1 in, 8 out]
  n117 = mathscript code="TL=abs(tl);\nvswr=(1+TL)/(1-TL);"("tl"=w115) -> ("??"=→"?":errorcluster, "vswr"=→"Ideal VSWR":dbl)  [unwired: 1 in]
  n118 = mathscript code="vmax=voutfi(1);\nvmin=voutfi(1);\nfor q=1:1:lenfin2\n   if (voutfi(q)>vmax)\n       vmax=voutfi(q);\n   end\n   if (voutfi(q)<vmin)\n       vmin=voutfi(q);\n   end\n   end\nvswrfi=vmax/vmin;"("lenfin2"=w120, "voutfi"=w118) -> ("vswrfi"=→"VSWR Meter":dbl)  [unwired: 1 in, 1 out]
  n119 = Current VI's Path() -> (path=w10:path)
  n120 = Path To String(path=w10) -> (string=→"Current VI path 11":string)
  n121 = Strip Path(path=w10) -> (stripped path=w15:path, name=→"Stripped Path 11":string)
  n122 = Build Path(base path=w15, name or relative path="vsw_fin01.jpg") -> (appended path=w8:path)
  n123 = Path To String(path=w15) -> (string=→"Part Stripped 11":string)
  n124 = Path To String(path=w8) -> (string=→"New Path for Picture 11":string)
  n125 = call <vilib>:"Read JPEG File.vi"("path to JPEG file"=path "C:/Program Files/Apache Software Foundation/Apache2.2/htdocs/exp1/vsw_fin01.jpg") -> ("image data"=w56:T3)  [unwired: 1 in, 9 out]
  n126 = call <vilib>:"Draw Flattened Pixmap.vi"("image data"=w56) -> ()  [unwired: 1 in, 8 out]
  n127 = feedback #7("2.TECNIQUE USED TO CALCULATE VSWR") -> (w144:bool)
  n128 = And(x=w144, y=FALSE) -> (x .and. y?=w142:bool)
  n129 = Wait For Front Panel Activity(3:w142) -> ()  [unwired: 3 out]
  n130 = call "Display Message to User8"("Enable"=w144) -> ("error out"=→"error out":errorcluster, "CLOSE"=w146:bool)  [unwired: 2 in, 7 out]
  n131 = feedback #8("1.TECNIQUE USED TO CALCULATE VSWR") -> (w150:bool)
  n132 = And(x=w150, y=FALSE) -> (x .and. y?=w148:bool)
  n133 = Wait For Front Panel Activity(3:w148) -> ()  [unwired: 3 out]
  n134 = call "Display Message to User7"("Enable"=w150) -> ("error out"=→"error out":errorcluster, "CLOSE"=w152:bool)  [unwired: 2 in, 7 out]
